vi "RIMAS Detector Update FITS Header.vi"(8 "Error In":errorcluster, 11 "Detector Config":T1={"Detector"=0, "Offsets"=[[0, 0, 0, 0, 0, 0, 0, 0, 0, 0, 0, 0, 0, 0, 0, 0, 0, 0, 0, 0, 0, 0, 0, 0, 0, 0, 0, 0, 0, 0, 0, 0]], "Detector Computer"={"Machine"="192.168.121.11", "Password"="", "FITS File Path"="", "Port"=44444, "Header Path"="", "Name"=""}, "FITS hdr template0"=path "", "FITS hdr template1"=path "", "FITS Data File Path"=path "", "FITS Detector Settings"={"Exp Time Short"=0.0, "# of Frames"=0.0, "Exp Time Long"=0.0, "# of Groups"=0.0, "Object Name"="", "Object"="", "Obs Type"="", "Image Type"="", "Observer"="", "Observer Affiliation"=""}, "Sim Folder"=path "", "Integration Mode"=enum."SSR", "Integration Time"=0.0, "Frame Int Time"=0.0} {"Offsets" format="%04x"; "Detector" items=["0", "1", "2"]}) -> (0 "Error Out":errorcluster, 3 "Files":path[](array[path]))   [LabVIEW 2022 SP3]
uses:
  RIMAS Detector Config.ctl
  RIMAS Detector Server Config.ctl
  RIMAS Observation Config.ctl
  Detector enum Detector Integration Mode.ctl
  <vilib>/Utility/error.llb/Trim Whitespace One-Sided.vi
panel:
  out "text":string[](array[string])
  out "Array":string[](array[string])
  out "fits hdr out":string[](array[string])
  # "C:\\Users\\shutters\\Documents\\header1.dat"
  # "sec"
  # "sec"
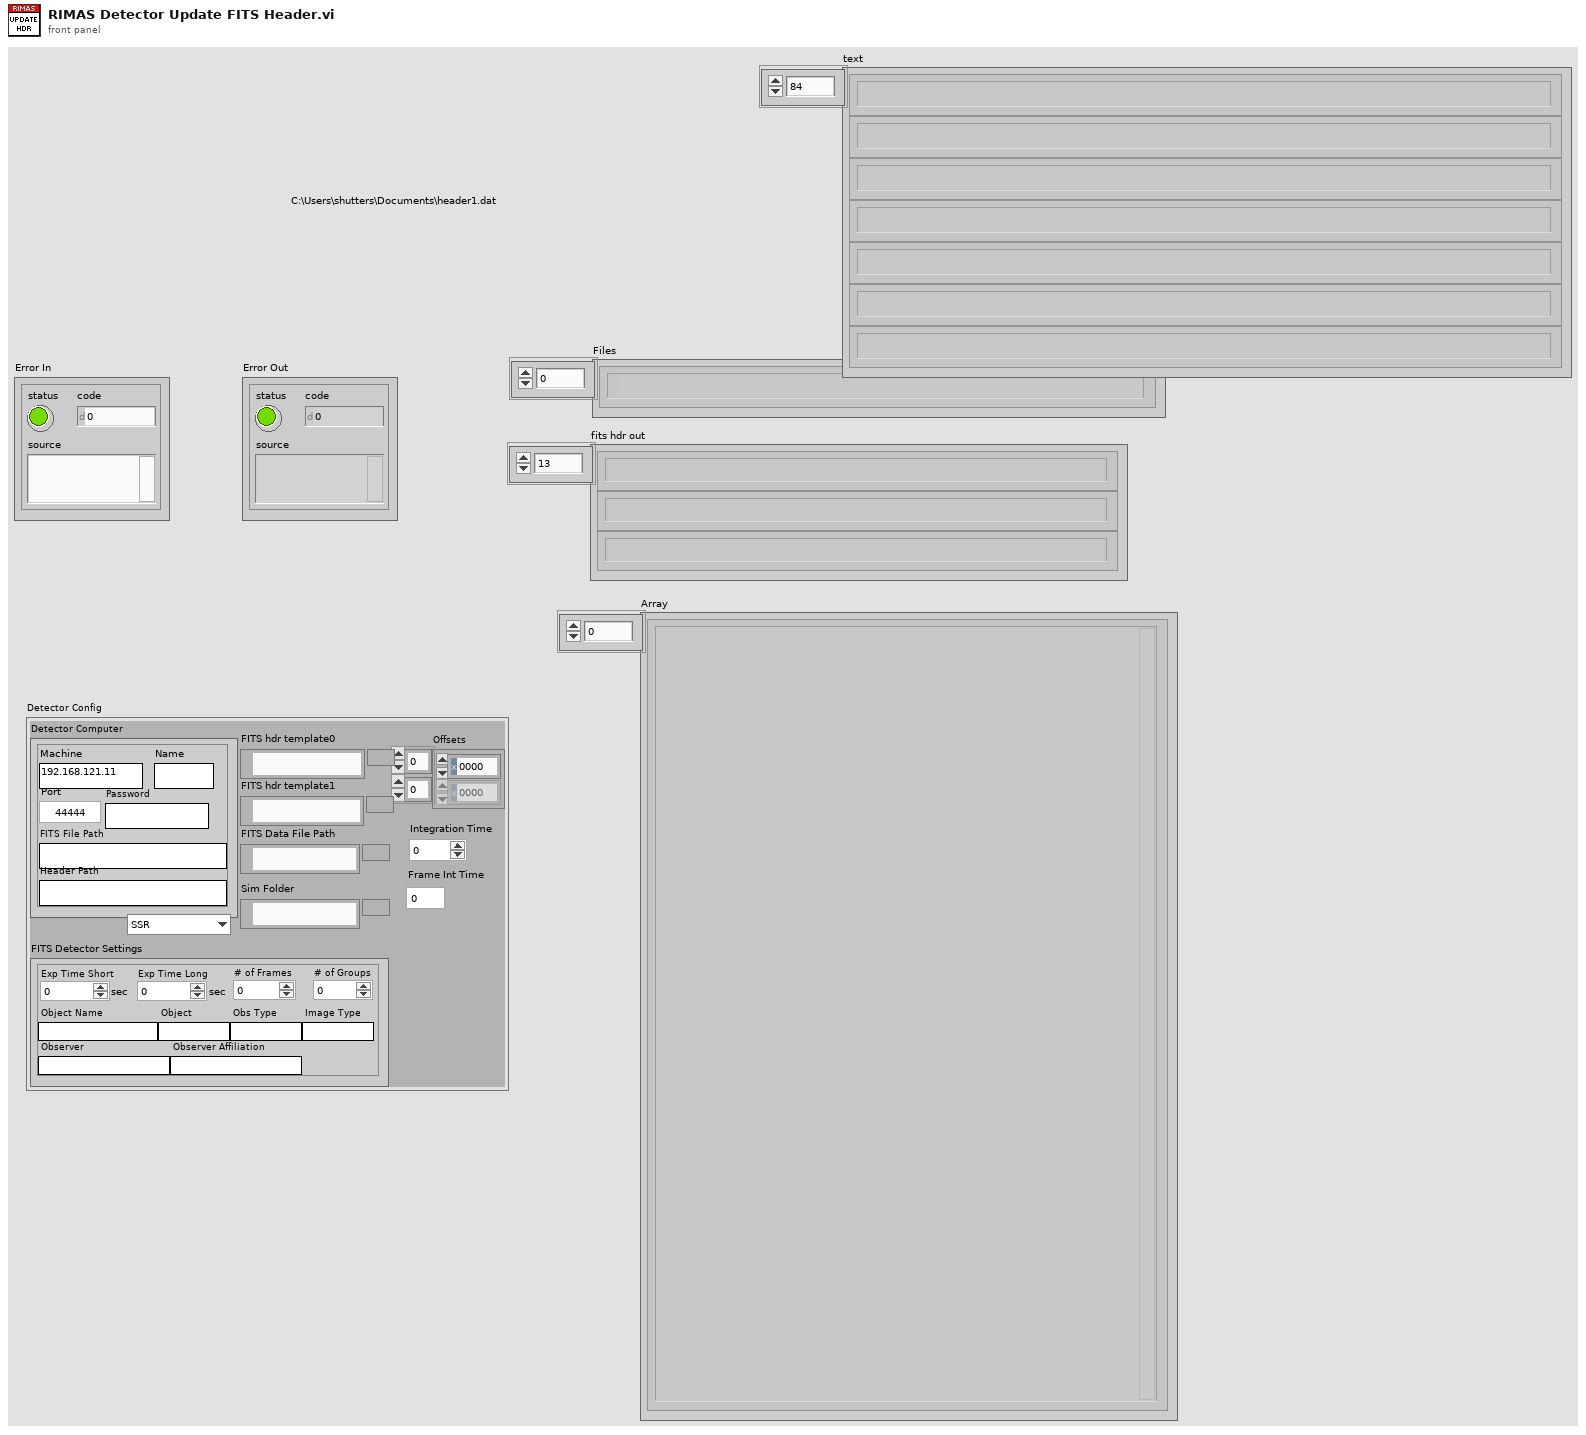
[diagram p1: front panel]
types:
  T1 = typedef "RIMAS Detector Config.ctl" = cluster{"Detector":u16, "Offsets":u16[][], "Detector Computer":T2, "FITS hdr template0":path, "FITS hdr template1":path, "FITS Data File Path":path, "FITS Detector Settings":T3, "Sim Folder":path, "Integration Mode":T4, "Integration Time":dbl, "Frame Int Time":dbl}
  T2 = typedef "RIMAS Detector Server Config.ctl" = cluster{"Machine":string, "Password":string, "FITS File Path":string, "Port":u16, "Header Path":string, "Name":string}
  T3 = typedef "RIMAS Observation Config.ctl" = cluster{"Exp Time Short":dbl, "# of Frames":dbl, "Exp Time Long":dbl, "# of Groups":dbl, "Object Name":string, "Object":string, "Obs Type":string, "Image Type":string, "Observer":string, "Observer Affiliation":string}
  T4 = typedef "Detector enum Detector Integration Mode.ctl" = enum16{"SSR", "CDS", "MEAN", "MEDIAN", "MODE", "MIIN", "MAX"}
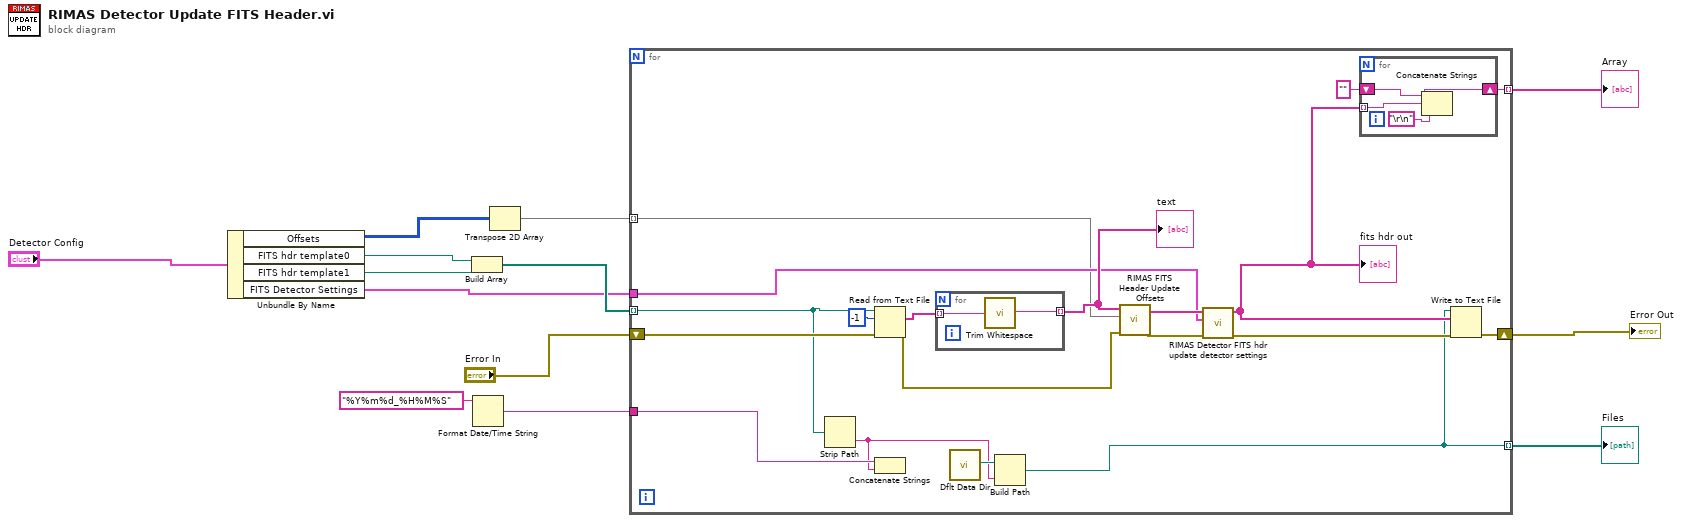
[diagram p0: block diagram]
diagram:
  n1 = Unbundle By Name("Detector Config") -> ("Offsets"=w2:u16[][], "FITS hdr template0"=w5:path, "FITS hdr template1"=w8:path, "FITS Detector Settings"=w3:T3)
  n2 = Build Array(w5, w8) -> (w9:path[])
  n3 = Format Date/Time String(time format string (%c)="%Y%m%d_%H%M%S") -> (date/time string=w12:string)  [unwired: 2 in]
  n4 = Transpose 2D Array(2D array=w2) -> (transposed array=w1:u16[][])
  n5 = for {
    tunnel: w12 -> [w29]
    tunnel: [w16] -> w7 mode=indexing
    shift-right: [w27] -> w10
    shift-left: "Error In" -> [w28]
    tunnel: w9 -> [w19] mode=indexing
    tunnel: [w20] -> w6 mode=indexing
    tunnel: w1 -> [w14] mode=indexing
    tunnel: w3 -> [w15]
    n6 = Strip Path(path=w19) -> (name=w23:string)  [unwired: 1 out]
    n7 = Read from Text File(file (use dialog)=w19, count=-1, error in=w28) -> (text=w18:string[], error out=w31:errorcluster)  [unwired: 1 in, 2 out]
    n8 = Concatenate Strings(w29, w23) -> ()  [unwired: 1 out]
    n9 = for {
      tunnel: w18 -> [w33] mode=indexing
      tunnel: [w34] -> w17 mode=indexing
      n10 = call <vilib>:"Trim Whitespace.vi"("string"=w33) -> ("trimmed string"=w34:string)  [unwired: 1 in]
    }
    "text" <- w17
    n11 = call <vilib>:"Dflt Data Dir.vi"() -> ("App:Default Data Directory"=w30:path)
    n12 = Build Path(base path=w30, name or relative path=w23) -> (appended path=w16:path)
    n13 = call "RIMAS FITS Header Update Offsets.vi"("Error In"=w31, "Offsets"=w14, "header file"=w17) -> ("Error Out"=w26:errorcluster, "updated hdr file"=w25:string[])  [unwired: 7 in]
    n14 = call "RIMAS Detector FITS hdr update detector settings.vi"("Error In"=w26, "FITS Detector Settings"=w15, "fits hdr"=w25) -> ("Error Out"=w24:errorcluster, "fits hdr out"=w22:string[])  [unwired: 7 in]
    "fits hdr out" <- w22
    n15 = for {
      shift-right: [w37] -> w20
      shift-left: "" -> [w38]
      tunnel: w22 -> [w36] mode=indexing
      n16 = Concatenate Strings(w38, w36, "\r\n") -> (w37:string)
    }
    n17 = Write to Text File(file (use dialog)=w16, text=w22, error in=w24) -> (error out=w27:errorcluster)  [unwired: 1 in, 2 out]
  }
  "Error Out" <- w10
  "Files" <- w7
  "Array" <- w6
